vi "main_modif.vi"() -> ()   [LabVIEW 2013]
panel:
  in  "?":bool=TRUE
  out "Waveform Chart":dbl(graph)
  in  "stop":bool
  out "DDP":string
  out "Porta livre?":bool=TRUE
  in  "baud rate (115200)":u32=115200
  in  "VISA Refnum in":refnum<visa-resource-name>="COM3"
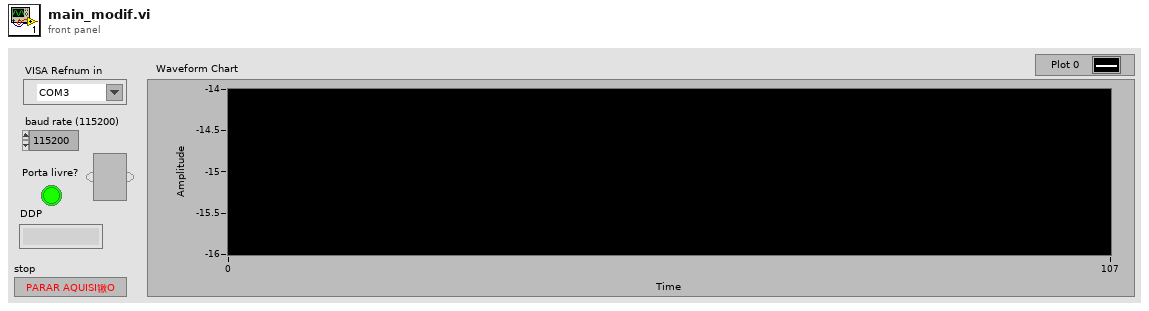
[diagram p1: front panel]
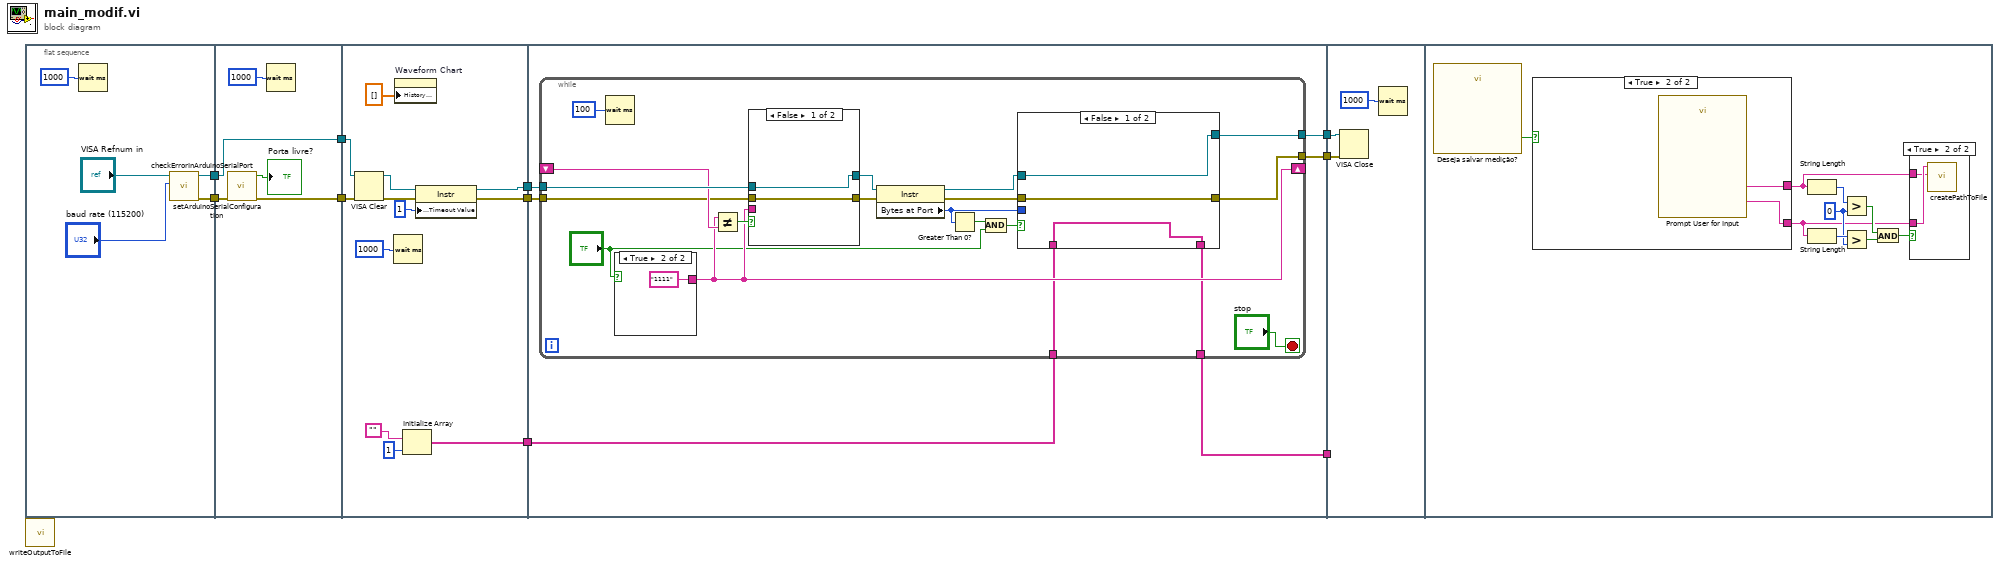
[diagram p0: block diagram]
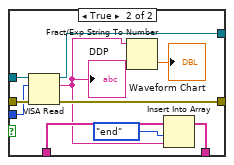
[diagram p2: hidden frame]
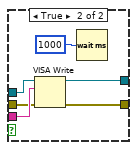
[diagram p3: hidden frame]
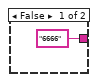
[diagram p4: hidden frame]
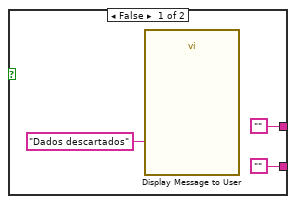
[diagram p6: hidden frame]
diagram:
  n1 = flat-sequence {
    tunnel: [w15] -> w8
    tunnel: [w14] -> w7
    tunnel: [w17] -> w10
    tunnel: [w20] -> w9
    tunnel: w8 -> [w20]
    tunnel: w7 -> [w18]
    tunnel: w10 -> [w32]
    tunnel: w9 -> [w31]
    tunnel: [w28] -> w4
    tunnel: [w26] -> w3
    tunnel: [w21] -> w2
    tunnel: [w38] -> w6
    tunnel: [w37] -> w5
    tunnel: w3 -> [w35]
    tunnel: w4 -> [w36]
    tunnel: w2 -> [w34]
    tunnel: [w33] -> w1
    tunnel: w6 -> [w82]
    tunnel: w5 -> [w81]
    tunnel: w1 -> [_]
    frame #0 {
      n2 = Wait (ms)(milliseconds to wait=u32 1000) -> ()  [unwired: 1 out]
      n3 = call "setArduinoSerialConfiguration.vi"("baud rate (9600)"="baud rate (115200)", "VISA Refnum in"="VISA Refnum in") -> ("error out"=w14:errorcluster, "VISA Refnum out"=w15:refnum<visa-resource-name>)  [unwired: 8 in]
    }
    frame #1 {
      n4 = call "checkErrorInArduinoSerialPort.vi"("error in (no error)"=w18) -> ("error out"=w17:errorcluster, "Porta livre?"=→"Porta livre?":bool)  [unwired: 9 in]
      n5 = Wait (ms)(milliseconds to wait=u32 1000) -> ()  [unwired: 1 out]
    }
    frame #2 {
      n6 = VISA Clear(VISA resource name=w31, error in (no error)=w32) -> (VISA resource name out=w29:refnum<visa-resource-name>, error out=w27:errorcluster)
      n7 = Wait (ms)(milliseconds to wait=u32 1000) -> ()  [unwired: 1 out]
      n8 = property on="Waveform Chart" class="WFChart (strict)"("History Data"=dbl[] []) -> ()  [unwired: 2 in, 2 out]
      n9 = Initialize Array("", 1 ("dimension size")) -> (w21:string[])
      n10 = property class="Instr"(reference=w29, error in=w27, "General Settings:Timeout Value"=u32 1) -> (reference out=w28:refnum<visa-resource-name>, error out=w26:errorcluster)
    }
    frame #3 {
      n11 = while {
        tunnel: [w54] -> w38
        tunnel: [w56] -> w37
        tunnel: w36 -> [w52]
        tunnel: w35 -> [w48]
        shift-right: [w49] -> _
        shift-left: _ -> [w51]
        tunnel: w34 -> [w40]
        tunnel: [w39] -> w33
        stop <- "stop" stop-if-true
        n12 = Wait (ms)(milliseconds to wait=u32 100) -> ()  [unwired: 1 out]
        n13 = case shown="True" "?" {
          tunnel: ["6666" ("write buffer") "1111" ("write buffer")] -> w49
          frame False {
          }
          frame True {
          }
        }
        n14 = Not Equal?(x=w49, y=w51) -> (x != y?=w50:bool)
        n15 = case shown="False" w50 {
          tunnel: w52 -> [w71 w78]
          tunnel: [w71 w77] -> w46
          tunnel: w49 -> [_ w76]
          tunnel: w48 -> [w72 w75]
          tunnel: [w72 w74] -> w47
          frame False {
          }
          frame True {
            n16 = VISA Write(VISA resource name=w78, write buffer=w76, error in (no error)=w75) -> (VISA resource name out=w77:refnum<visa-resource-name>, error out=w74:errorcluster)  [unwired: 1 out]
            n17 = Wait (ms)(milliseconds to wait=u32 1000) -> ()  [unwired: 1 out]
          }
        }
        n18 = property class="Instr"(reference=w46, error in=w47) -> (reference out=w57:refnum<visa-resource-name>, error out=w55:errorcluster, "Bytes at Port"=w45:u32)
        n19 = Greater Than 0?(x=w45) -> (x > 0?=w43:bool)
        n20 = And(x=w43, y="?") -> (x .and. y?=w41:bool)
        n21 = case shown="False" w41 {
          tunnel: w57 -> [w60 w70]
          tunnel: [w60 w69] -> w56
          tunnel: w55 -> [w59 w68]
          tunnel: [w59 w67] -> w54
          tunnel: w45 -> [_ w65]
          tunnel: w40 -> [w58 w64]
          tunnel: [w58 w61] -> w39
          frame False {
          }
          frame True {
            n22 = VISA Read(VISA resource name=w70, byte count=w65, error in (no error)=w68) -> (VISA resource name out=w69:refnum<visa-resource-name>, read buffer=w63:string, error out=w67:errorcluster)  [unwired: 1 out]
            "DDP" <- w63
            n23 = Fract/Exp String To Number(string=w63) -> (number=→"Waveform Chart":dbl)  [unwired: 3 in, 1 out]
            n24 = Insert Into Array(array=w64, index=enum16{"start", "end", "current"}."end" ("from (0:start)"), new element=w63) -> (w61:string[])
          }
        }
      }
    }
    frame #4 {
      n25 = VISA Close(VISA resource name=w81, error in (no error)=w82) -> ()  [unwired: 1 out]
      n26 = Wait (ms)(milliseconds to wait=u32 1000) -> ()  [unwired: 1 out]
    }
    frame #5 {
      w88 = 0 ("y")
      n27 = call "Deseja salvar medição?"() -> ("SIM"=w92:bool)  [unwired: 18 in, 1 out]
      n28 = case shown="True" w92 {
        tunnel: ["" w99] -> w91
        tunnel: ["" w98] -> w84
        frame False {
          n29 = call "Display Message to User"("Message"="Dados descartados") -> ()  [unwired: 9 in, 2 out]
        }
        frame True {
          n30 = call "Prompt User for Input"() -> ("Nome"=w98:string, "Pasta"=w99:string)  [unwired: 16 in, 2 out]
        }
      }
      n31 = String Length(string=w91) -> (length=w90:i32)
      n32 = String Length(string=w84) -> (length=w89:i32)
      n33 = Greater?(x=w90, y=w88) -> (0:w86:bool)
      n34 = Greater?(x=w89, y=w88) -> (0:w87:bool)
      n35 = And(x=w86, y=w87) -> (x .and. y?=w85:bool)
      n36 = case shown="True" w85 {
        tunnel: w91 -> [_ w93]
        tunnel: w84 -> [_ w94]
        frame False {
        }
        frame True {
          n37 = call "createPathToFile.vi"("Pasta"=w93, "Nome"=w94) -> ()  [unwired: 9 in, 1 out]
        }
      }
    }
  }
  n38 = call "writeOutputToFile.vi"() -> ()  [unwired: 5 in, 1 out]
